vi "Get Image on PC.vi"(8 "error in (no error)":errorcluster, 10 "Cluster in":T2, 11 "Refnum in":T1) -> (0 "error out":errorcluster, 2 "Cluster out":T2, 3 "Refnum out":T1)   [LabVIEW 2015]
uses:
  Camera Network Settings.ctl
  <vilib>/vision/Image Controls.llb/IMAQ Image.ctl
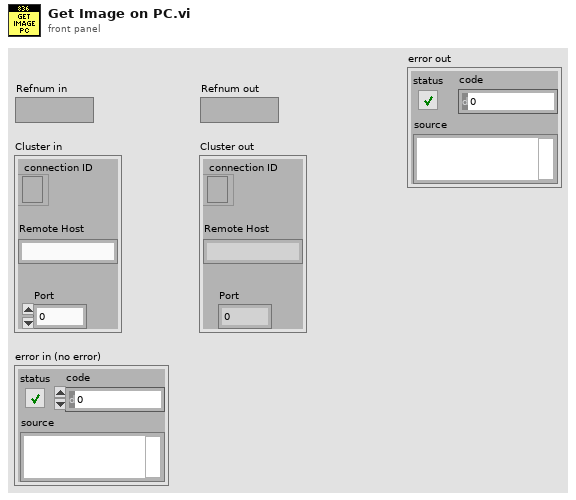
[diagram p1: front panel]
types:
  T1 = typedef "IMAQ Image.ctl" = refnum<image>
  T2 = typedef "Camera Network Settings.ctl" = cluster{"connection ID":refnum<k5>, "Port":u16, "Remote Host":string}
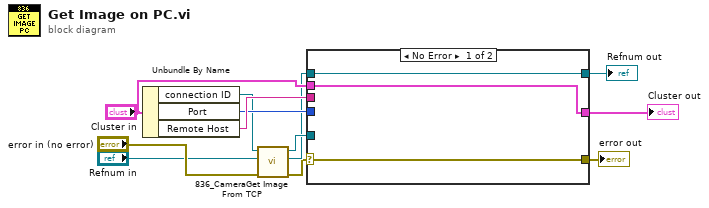
[diagram p0: block diagram]
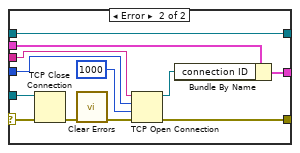
[diagram p2: hidden frame]
diagram:
  n1 = Unbundle By Name("Cluster in") -> ("connection ID"=w3:refnum<k5>, "Port"=w9:u16, "Remote Host"=w10:string)
  n2 = call "836_CameraGet Image From TCP.vi"("error in (no error)"="error in (no error)", "Image In"="Refnum in", "connection ID"=w3) -> ("error out"=w4:errorcluster, "Image Out"=w5:T1, "connection ID (dup)"=w7:refnum<k5>)  [unwired: 3 in, 3 out]
  n3 = case shown="No Error" w4 {
    selector: w4 -> [w13 w27]
    tunnel: w5 -> [w15 w25]
    tunnel: [w15 w25] -> w6
    tunnel: w7 -> [_ w26]
    tunnel: "Cluster in" -> [w14 w23]
    tunnel: [w14 w17] -> w11
    tunnel: w9 -> [_ w19]
    tunnel: w10 -> [_ w18]
    tunnel: [w13 w16] -> w1
    frame No Error {
    }
    frame Error {
      n4 = TCP Close Connection(connection ID=w26, error in (no error)=w27) -> (error out=w21:errorcluster)  [unwired: 1 in, 1 out]
      n5 = call <vilib>:"Clear Errors.vi"("error in (no error)"=w21) -> ("error out"=w20:errorcluster)  [unwired: 5 in, 1 out]
      n6 = TCP Open Connection(address=w18, remote port or service name=w19, timeout ms (60000)=1000, error in (no error)=w20) -> (connection ID=w22:refnum<k5>, error out=w16:errorcluster)  [unwired: 1 in]
      n7 = Bundle By Name(cluster=w23, "connection ID"=w22) -> (w17:T2)
    }
  }
  "Cluster out" <- w11
  "Refnum out" <- w6
  "error out" <- w1
